vi "ResonanceAnalyzer.vi"() -> ()   [LabVIEW 2015]
uses:
  <vilib>/imath/engines/lvmath2/RunTimeEngine/Managers/WorkSpace/UID Generator.vi
  <vilib>/imath/engines/lvmath2/RunTimeEngine/RangeToken/NIMS_Range.vi
  <instcachedir>/0/NIMS_Range_D919CC09935940E88F755EC1C6F49AC1.lvgen/NIMS_Range_D919CC09935940E88F755EC1C6F49AC1_000.vi
  <vilib>/imath/engines/lvmath2/RunTimeEngine/RunTimeType/NIMS_RunTimeType_From StrictType (excl LVString).vi
  <instcachedir>/0/NIMS_RunTimeType_From StrictType (excl LVString)_EB1C38A9BC5048DA9ABDA8F781E54D21.lvgen/NIMS_RunTimeType_From StrictType (excl LVString)_EB1C38A9BC5048DA9ABDA8F781E54D21_000.vi
  <vilib>/imathl/engines/lvmath/Functions/Error Handling/Create Error.vi
  <vilib>/imath/engines/lvmath2/RunTimeEngine/LocalVariableDefStatement/MC_LocalVariableDefStatement_Display.vi
  <vilib>/imath/engines/lvmath2/RunTimeEngine/ArithmeticOperatorToken/NIMS_ArithmeticOperator_plus.vi
  <instcachedir>/0/NIMS_ArithmeticOperator_plus_A4F2756F5ADB4A0090E0DBD7C10701C8.lvgen/NIMS_ArithmeticOperator_plus_A4F2756F5ADB4A0090E0DBD7C10701C8_004.vi
  <vilib>/imath/engines/lvmath2/RunTimeEngine/ArithmeticOperatorToken/NIMS_ArithmeticOperator_rightdiv.vi
  <instcachedir>/0/NIMS_ArithmeticOperator_rightdiv_E8FF7CD3D5774FA6AA728C3F0517CAD4.lvgen/NIMS_ArithmeticOperator_rightdiv_E8FF7CD3D5774FA6AA728C3F0517CAD4_000.vi
  <vilib>/imath/engines/lvmath2/RunTimeEngine/ErrorHandling/NIMS_Create Error From Enums.vi
  <vilib>/imath/engines/lvmath2/RunTimeEngine/BuiltInFunctions/randnormal/NIMS_randnormal(1,I32).vi
  <vilib>/imath/engines/lvmath2/RunTimeEngine/ErrorHandling/NIMS_Error From Error Code.vi
  <vilib>/imath/engines/lvmath2/RunTimeEngine/Managers/SymbolTable/Clear UID.vi
  <vilib>/imath/engines/lvmath2/RunTimeEngine/NodeEndStatement/NIMS_NodeEndStatement_Output.vi
  <instcachedir>/0/NIMS_NodeEndStatement_Output_53EC0D466D134D7ABD903AC30B43404B.lvgen/NIMS_NodeEndStatement_Output_53EC0D466D134D7ABD903AC30B43404B_005.vi
  <vilib>/imath/engines/lvmath2/RunTimeEngine/ErrorHandling/NIMS_Finalize Error.vi
  <vilib>/Utility/file.llb/Read Delimited Spreadsheet (DBL).vi
  <vilib>/imath/engines/lvmath2/RunTimeEngine/Managers/SymbolTable/NIMS_WorkSpace.lvlib
panel:
  out "Results":T1={"Amplitude"=0.46420851943485414, "Center Freq"=660.7809764179497, "Q"=30.036998679596458, "Array[3]"=0.0, "Array[4]"=0.0, "Array[5]"=0.0, "Array[6]"=0.0, "Array[7]"=0.0, "Array[8]"=0.0}
  out "XY Graph":cluster{"Array":dbl[], "x":dbl[]}[](graph)=[{"Array"=[580.0, 590.0, 600.0, 610.0, 620.0, 630.0, 640.0, 650.0, 660.0, 670.0, 680.0, 690.0, 700.0, 710.0, 720.0, 730.0, 740.0], "x"=[0.09192846321567942, 0.09491831063496878, 0.10205869245905823, 0.11535860616795962, 0.13928360536656795, 0.15073010441631318, 0.20179016711531975, 0.32591173631348447, 0.45893375327940794, 0.37931498497368193, 0.21269143432035517, 0.1451443049430261, 0.11172490653048396, 0.09321804703416083, 0.08229055663189361, 0.07599762143610374, 0.07320656005152644]}, {"Array"=[580.0, 590.0, 600.0, 610.0, 620.0, 630.0, 640.0, 650.0, 660.0, 670.0, 680.0, 690.0, 700.0, 710.0, 720.0, 730.0, 740.0], "x"=[0.058620187588099594, 0.06733648770205389, 0.07879694905748195, 0.09451035560826002, 0.11728677891959283, 0.15289227444934103, 0.21443858143773475, 0.3301764137935174, 0.4630414665881881, 0.3567840767693754, 0.233059435841523, 0.16663205524950947, 0.12869483090814024, 0.10469711977585133, 0.08827988178563753, 0.07638227098582054, 0.0673786670510282]}]
  in  "Tab Control":enum32{" Simulation", "Experiment"}(tab)=enum."Experiment"
  in  "Cluster":T2={"Q"=30.0, "Center Frequency"=600.0, "Start Frequency"=400.0, "End Frequency"=800.0, "df "=5.0, "Noise Level"=0.01}
  in  "Path":path=path "C:/Users/jamism2/Desktop/PHYS434jampet/week5/SinglePeak.txt"
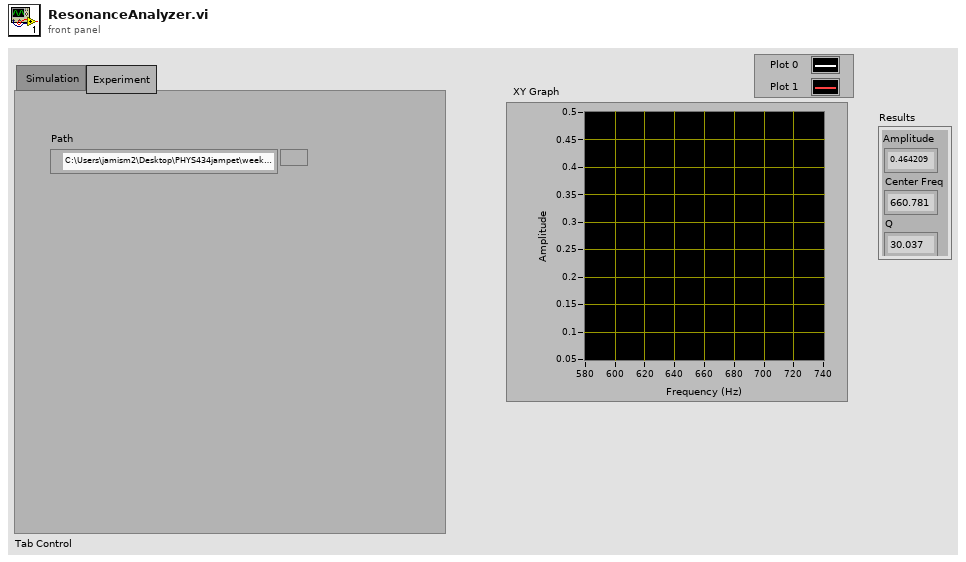
[diagram p1: front panel]
types:
  T1 = cluster{"Amplitude":dbl, "Center Freq":dbl, "Q":dbl, "Array[3]":dbl, "Array[4]":dbl, "Array[5]":dbl, "Array[6]":dbl, "Array[7]":dbl, "Array[8]":dbl}
  T2 = cluster{"Q":dbl, "Center Frequency":dbl, "Start Frequency":dbl, "End Frequency":dbl, "df ":dbl, "Noise Level":dbl}
  T3 = cluster{"Array[0]":dbl, "Array[1]":dbl, "Array[2]":dbl, "Array[3]":dbl, "Array[4]":dbl, "Array[5]":dbl, "Array[6]":dbl, "Array[7]":dbl, "Array[8]":dbl}
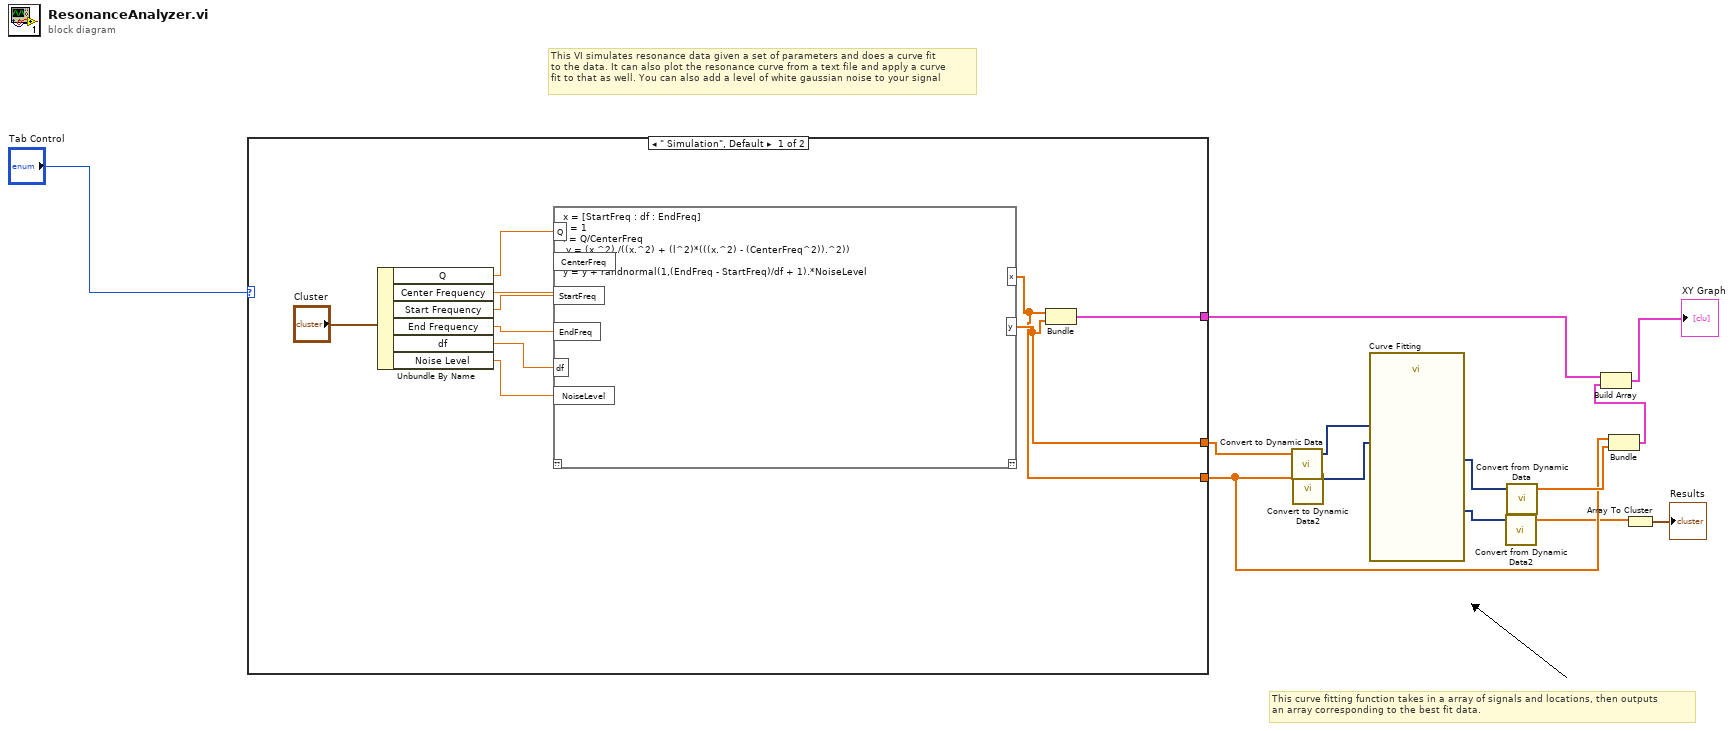
[diagram p0: block diagram]
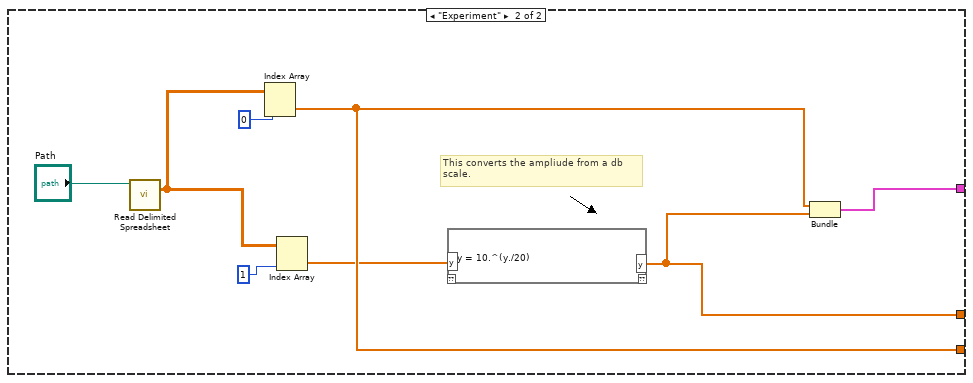
[diagram p2: hidden frame]
diagram:
  # "This curve fitting function takes in a array of signals and locations, then outputs \nan array corresponding to the best fit data."
  # "This VI simulates resonance data given a set of parameters and does a curve fit \nto the data. It can also plot the resonance curve from a text file and apply a curve\nfit to that as well. You can also add a level of white gaussian noise to your signal"
  n1 = case shown="\" Simulation\", Default" "Tab Control" {
    tunnel: [w17 w208] -> w7
    tunnel: [w16 w204] -> w11
    tunnel: [w15 w207] -> w4
    frame " Simulation", Default {
      n2 = Unbundle By Name("Cluster") -> ("Q"=w22:dbl, "Center Frequency"=w21:dbl, "Start Frequency"=w20:dbl, "End Frequency"=w19:dbl, "df"=w18:dbl, "Noise Level"=w14:dbl)
      n3 = mathscript code="x = [StartFreq : df : EndFreq]\nr = 1\nl = Q/CenterFreq\n y = (x.^2)./((x.^2) + (l^2)*(((x.^2) - (CenterFreq^2)).^2))\n\ny = y + randnormal(1,(EndFreq - StartFreq)/df + 1).*NoiseLevel"("Q"=w22, "CenterFreq"=w21, "StartFreq"=w20, "EndFreq"=w19, "df"=w18, "NoiseLevel"=w14) -> ("y"=w16:dbl[], "x"=w15:dbl[])  [unwired: 1 in, 1 out]
      n4 = Bundle("x"=w15, "y"=w16) -> (w17:cluster{"x":dbl[], "y":dbl[]})  [unwired: 1 in]
    }
    frame "Experiment" {
      # "This converts the ampliude from a db\nscale."
      n5 = call-poly <vilib>:"Read Delimited Spreadsheet.vi"("file path (dialog if empty)"="Path") -> ("all rows"=w209:dbl[][])  [unwired: 9 in, 5 out]
      n6 = Index Array(array=w209, index (col)=0) -> (element=w207:dbl[])  [unwired: 1 in]
      n7 = Index Array(array=w209, index (col)=1) -> (element=w205:dbl[])  [unwired: 1 in]
      n8 = mathscript code="y = 10.^(y./20)"("y"=w205) -> ("y"=w204:dbl[])  [unwired: 1 in, 1 out]
      n9 = Bundle("all rows"=w207, "y"=w204) -> (w208:cluster{"all rows":dbl[], "y":dbl[]})  [unwired: 1 in]
    }
  }
  n10 = call "Convert to Dynamic Data"("Array"=w11) -> ("Dynamic Data Type"=w10:dynamicdata)  [unwired: 3 in]
  n11 = call "Convert to Dynamic Data2"("Array"=w4) -> ("Dynamic Data Type"=w12:dynamicdata)  [unwired: 3 in]
  n12 = call "Curve Fitting"("Locations"=w12, "Signals"=w10) -> ("best fit"=w9:dynamicdata, "non-linear coefficients"=w3:dynamicdata)  [unwired: 5 in, 3 out]
  n13 = call "Convert from Dynamic Data2"("Dynamic Data Type"=w3) -> ("Array"=w2:dbl[])  [unwired: 3 in]
  n14 = call "Convert from Dynamic Data"("Dynamic Data Type"=w9) -> ("Array"=w5:dbl[])  [unwired: 3 in]
  n15 = Bundle("all rows"=w4, "Array"=w5) -> (w8:cluster{"all rows":dbl[], "Array":dbl[]})  [unwired: 1 in]
  n16 = Build Array(w7, w8) -> (→"XY Graph":cluster{"all rows":dbl[], "Array":dbl[]}[])
  n17 = Array To Cluster(array=w2) -> (cluster=→"Results":T3)
